vi "Configure Device.vi"(8 "error in":errorcluster, 11 "Device in":refnum<class "Configurable Device.lvclass">) -> (0 "error out":errorcluster, 3 "Device out":refnum<class "Configurable Device.lvclass">, 4 "SP":dbl, 5 "Settable?":bool)   [LabVIEW 2017, in "Configurable Device.lvclass"]
doc: "This is the configuration method for the Device object. The one parameter that all should have in common and is not dependent on the configuration of the device is the label which is read from the ini file. All devices that use this class should have this in their configuration."
uses:
  Configurable Device.lvclass
  <vilib>/MSR Consulting, LLC/General Reuse/Session APIs/File Access/Config Data/Config Data.lvclass
  Configurable Device.lvclass/Configurable Device.ctl
  <vilib>/MSR Consulting, LLC/General Reuse/Session APIs/File Access/Config Data/Config Data.lvclass/Config Data.ctl
  <vilib>/MSR Consulting, LLC/General Reuse/Session APIs/File Access/Config Data/Accessors/Read Ref.vi
  <vilib>/Utility/config.llb/Read Key (String).vi
  <vilib>/Utility/config.llb/NI_LVConfig.lvlib
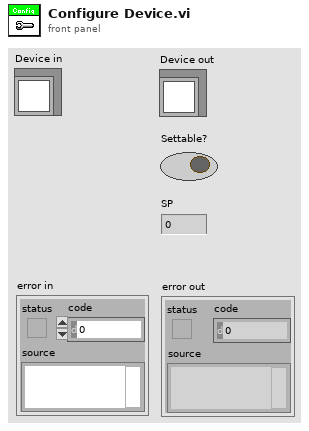
[diagram p1: front panel]
types:
  T1 = typedef "Session - Root.lvclass/Session Handle.ctl" = refnum<data-value>
  T2 = typedef "NI_LVConfig.lvlib/Config Data RefNum.ctl" = refnum<k1>
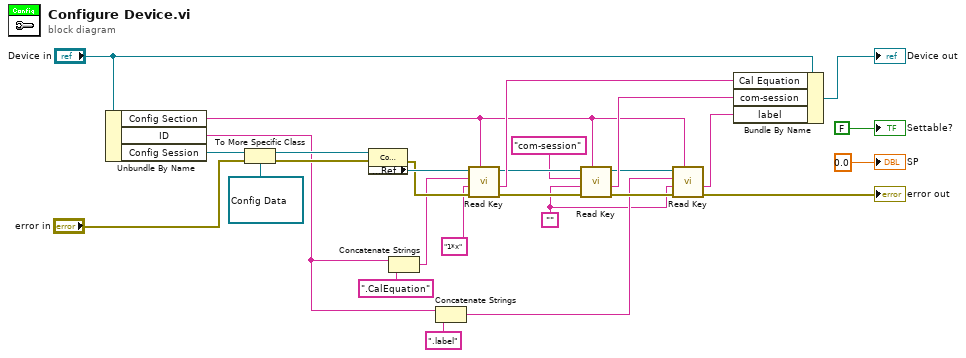
[diagram p0: block diagram]
diagram:
  w2 = ""
  n1 = Unbundle By Name("Device in") -> ("Config Section"=w4:string, "ID"=w7:string, "Config Session"=w28:T1)
  n2 = To More Specific Class(target class=refnum<data-value> refnum ("Config Session"), reference=w28, error in="error in") -> (specific class reference=w26:refnum<data-value>, error out=w25:errorcluster)
  n3 = property class="Config Data"(reference=w26, error in=w25) -> (error out=w20:errorcluster, "Accessors:Ref"=w21:T2)  [unwired: 1 out]
  n4 = Concatenate Strings(w7, ".CalEquation" ("ID")) -> (w19:string)
  n5 = Concatenate Strings(w7, ".label" ("string")) -> (w5:string)
  n6 = call-poly <vilib>:"Read Key.vi"("section"=w4, "error in (no error)"=w20, "default value"="1*x", "key"=w19, "refnum"=w21) -> ("error out"=w12:errorcluster, "value"=w16:string, "refnum out"=w13:T2)  [unwired: 3 in, 1 out]
  n7 = call-poly <vilib>:"Read Key.vi"("section"=w4, "error in (no error)"=w12, "default value"=w2, "key"="com-session", "refnum"=w13) -> ("error out"=w8:errorcluster, "value"=w10:string, "refnum out"=w9:T2)  [unwired: 3 in, 1 out]
  n8 = call-poly <vilib>:"Read Key.vi"("section"=w4, "error in (no error)"=w8, "default value"=w2, "key"=w5, "refnum"=w9) -> ("error out"=→"error out":errorcluster, "value"=w3:string)  [unwired: 3 in, 2 out]
  n9 = Bundle By Name(cluster="Device in", "Cal Equation"=w16, "com-session"=w10, "label"=w3) -> (→"Device out":refnum<class "Configurable Device.lvclass">)
  "SP" <- 0.0 ("SP")
  "Settable?" <- FALSE ("Settable?")
